vi "Update Metadata using table names.vi"(8 "error in":errorcluster) -> (0 "error out":errorcluster)   [LabVIEW 2010]
uses:
  <vilib>/addons/database/Connection.llb/DB Tools Open Connec (Path).vi
  <vilib>/addons/database/Connection.llb/Conn Execute.vi
  <vilib>/addons/database/Recordset.llb/Rec Destroy - Connection.vi
  <vilib>/addons/database/NI_Database_API.lvlib
panel:
  out "tableNamesOut":string[](array[string])
  in  "tableNamesIn":string[](array[string])
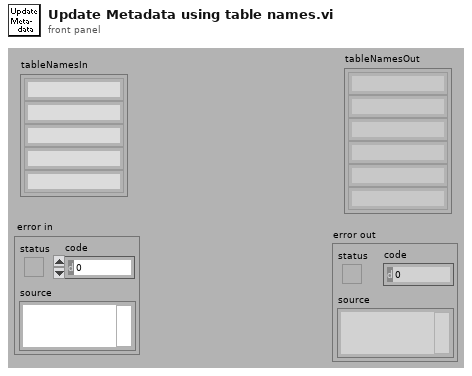
[diagram p1: front panel]
types:
  T1 = typedef "NI_Database_API.lvlib/Conn ObjectReference.ctl" = refnum<k1>
  T2 = typedef "NI_Database_API.lvlib/Rec ObjectReference.ctl" = refnum<k1>
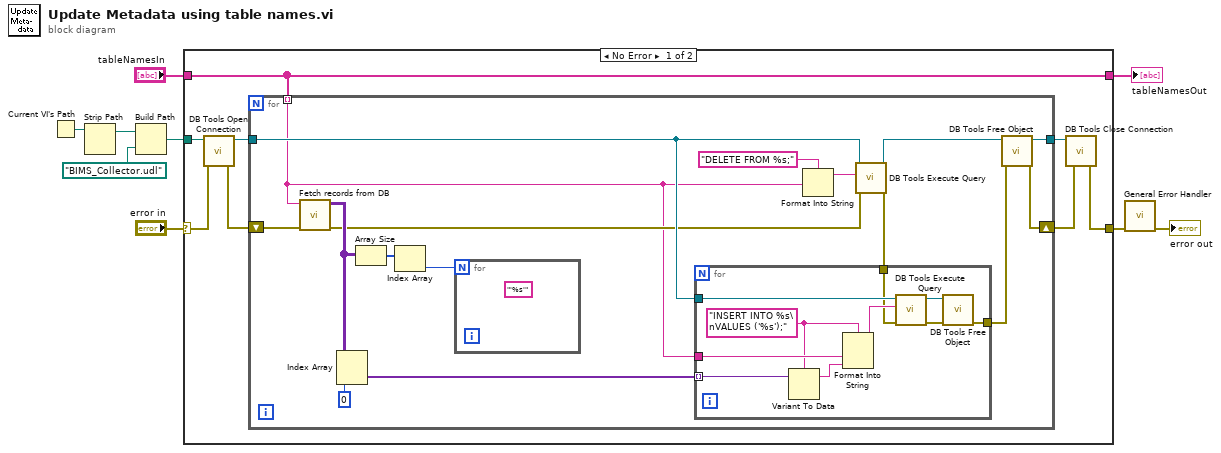
[diagram p0: block diagram]
diagram:
  n1 = Current VI's Path() -> (path=w8:path)
  n2 = Strip Path(path=w8) -> (stripped path=w7:path)  [unwired: 1 out]
  n3 = Build Path(base path=w7, name or relative path=path "BIMS_Collector.udl" ("connectString")) -> (appended path=w9:path)
  n4 = case shown="No Error" "error in" {
    selector: "error in" -> [w12 w44]
    tunnel: w9 -> [w15 _]
    tunnel: [w10 w44] -> w4
    tunnel: "tableNamesIn" -> [w11 w45]
    tunnel: [w11 w45] -> w2
    frame No Error {
      n5 = call-poly <vilib>:"DB Tools Open Connection.vi"("error in (no error)"=w12, "connection information"=w15) -> ("error out"=w17:errorcluster, "connection reference"=w16:T1)  [unwired: 3 in, 3 out]
      n6 = for {
        shift-right: [w32] -> w13
        shift-left: w17 -> [w20]
        tunnel: w16 -> [w30]
        tunnel: [w33] -> w14
        tunnel: w11 -> [w18] mode=indexing
        n7 = call "Fetch records from DB.vi"("error in"=w20, "Query"=w18) -> ("error out"=w19:errorcluster, "recordset data"=w21:variant[][])  [unwired: 4 out]
        n8 = Index Array(array=w21, index (col)=0 ("disabled index (col)")) -> (element=w31:variant[])  [unwired: 1 in]
        n9 = Array Size(array=w21) -> (size(s)=w23:i32[])
        n10 = Index Array(array=w23) -> (element=w22:i32)  [unwired: 1 in]
        n11 = for {
          N: w22 -> [_]
          (unwired) "'%s'" ("SQL query")
        }
        n12 = Format Into String(format string="DELETE FROM %s;" ("SQL query"), w18) -> (resulting string=w26:string)  [unwired: 2 in, 1 out]
        n13 = call-poly <vilib>:"DB Tools Execute Query.vi"("error in (no error)"=w19, "SQL query"=w26, "connection reference"=w30) -> ("error out"=w24:errorcluster, "recordset reference"=w29:T2)  [unwired: 1 in, 4 out]
        n14 = for {
          tunnel: w31 -> [w36] mode=indexing
          tunnel: w30 -> [w42]
          tunnel: [w39] -> w28
          tunnel: w24 -> [w38]
          tunnel: w18 -> [w37]
          w34 = "INSERT INTO %s\nVALUES ('%s');" ("SQL query")
          n15 = Variant To Data(Variant=w36, type=w34) -> (data=w35:string)  [unwired: 1 in, 1 out]
          n16 = Format Into String(format string=w34, w37, w35) -> (resulting string=w43:string)  [unwired: 2 in, 1 out]
          n17 = call-poly <vilib>:"DB Tools Execute Query.vi"("error in (no error)"=w38, "SQL query"=w43, "connection reference"=w42) -> ("error out"=w41:errorcluster, "recordset reference"=w40:T2)  [unwired: 1 in, 4 out]
          n18 = call-poly <vilib>:"DB Tools Free Object.vi"("error in (no error)"=w41, "recordset reference"=w40) -> ("error out"=w39:errorcluster)  [unwired: 9 out]
        }
        n19 = call-poly <vilib>:"DB Tools Free Object.vi"("error in (no error)"=w28, "recordset reference"=w29) -> ("error out"=w32:errorcluster, "connection reference"=w33:T1)  [unwired: 8 out]
      }
      n20 = call <vilib>:"DB Tools Close Connection.vi"("error in (no error)"=w13, "connection reference"=w14) -> ("error out"=w10:errorcluster)  [unwired: 5 out]
    }
    frame Error {
    }
  }
  "tableNamesOut" <- w2
  n21 = call <vilib>:"General Error Handler.vi"("error in (no error)"=w4) -> ("error out"=→"error out":errorcluster)  [unwired: 1 in, 13 out]
